vi "Buffer Calculation.vi"(10 "Buffer":dbl, 11 "Input":dbl) -> (1 "-Buffer":dbl, 3 "+Buffer":dbl)   [LabVIEW 2017]
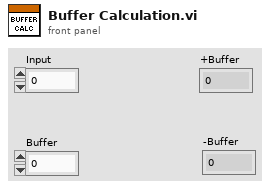
[diagram p1: front panel]
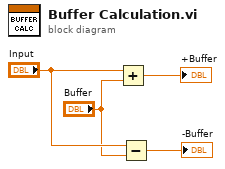
[diagram p0: block diagram]
diagram:
  n1 = Add(x="Input", y="Buffer") -> (x+y=→"+Buffer":dbl)
  n2 = Subtract(x="Input", y="Buffer") -> (x-y=→"-Buffer":dbl)
